vi "Kontrola poprawnego zakresu współrzędnej.vi"(8 "Sekundy":dbl, 9 "Minuty":dbl, 10 "Stopnie":dbl, 11 "Format współrzędnych":u16(ring) items=["D", "DM", "DMS"]) -> (0 "error constant":errorcluster)   [LabVIEW 2012, in "Biblioteka moduł map v3.lvlib" / "Konwersja wsp.lvlib" / "Obsługa błędów.lvlib"]
doc: "SubVI ma za zadanie sprawdzić poprawność zakresu wpisanych stopni, minut i sekund. Oraz czy nie wpisano dodatkowo minut i sekund, gdy wpisano maksymalną wartość stopni."
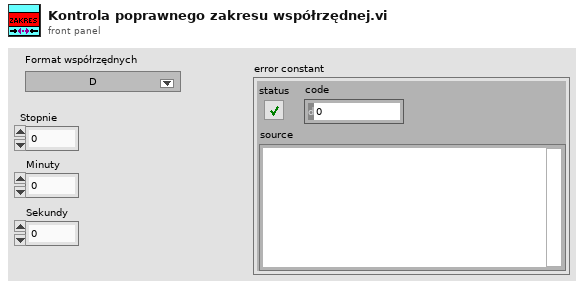
[diagram p1: front panel]
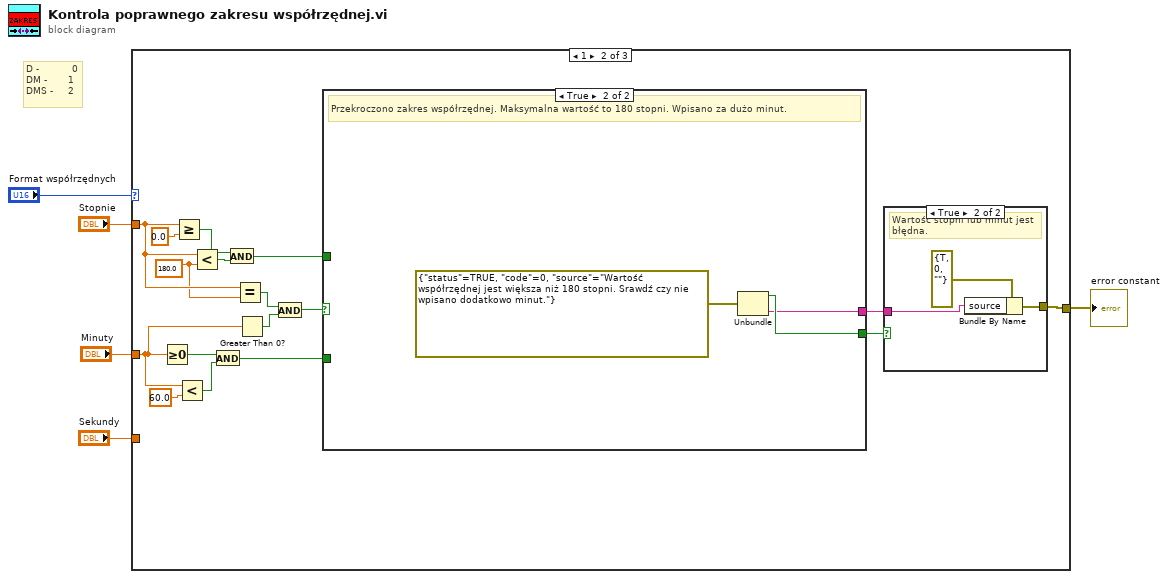
[diagram p0: block diagram]
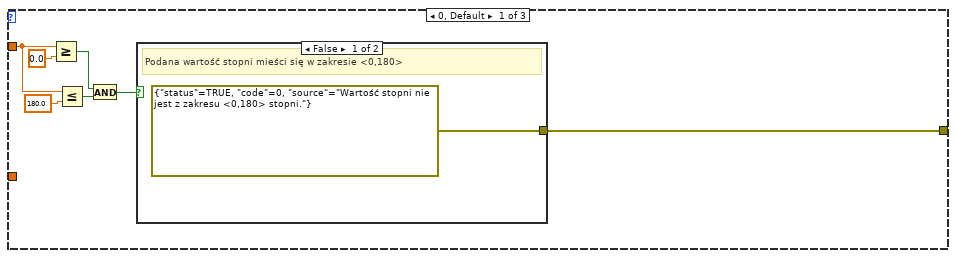
[diagram p2: hidden frame]
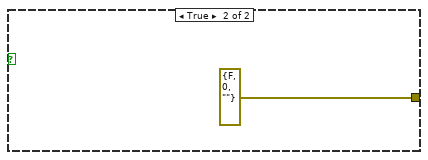
[diagram p3: hidden frame]
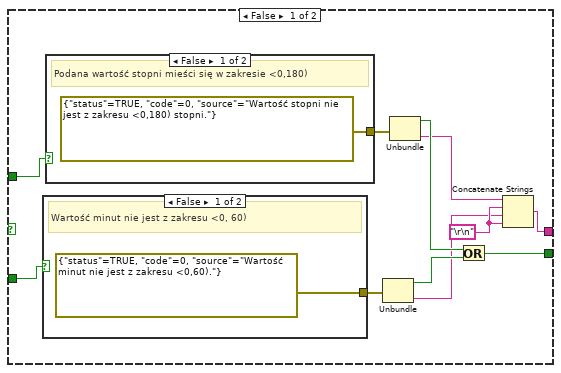
[diagram p4: hidden frame]
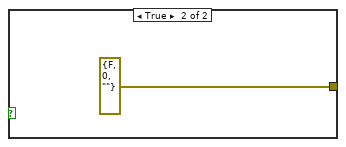
[diagram p5: hidden frame]
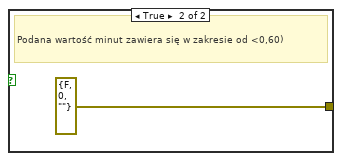
[diagram p6: hidden frame]
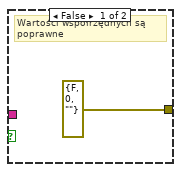
[diagram p7: hidden frame]
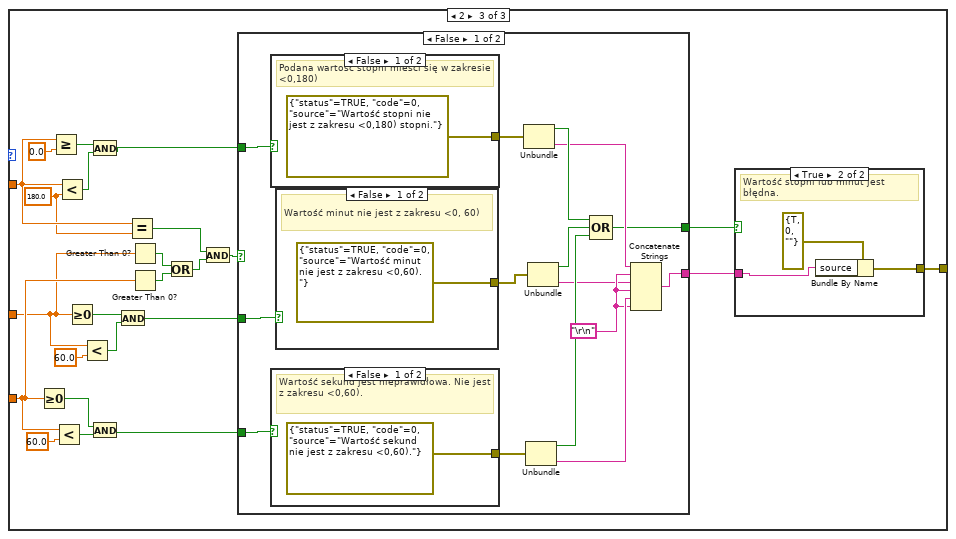
[diagram p8: hidden frame]
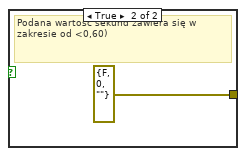
[diagram p9: hidden frame]
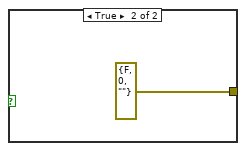
[diagram p10: hidden frame]
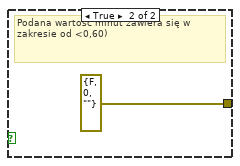
[diagram p11: hidden frame]
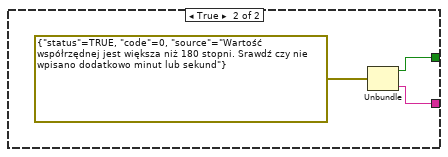
[diagram p12: hidden frame]
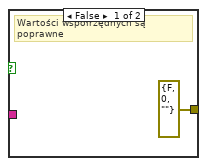
[diagram p13: hidden frame]
diagram:
  # "D -           0\nDM -       1\nDMS -     2"
  n1 = case shown="1" "Format współrzędnych" {
    tunnel: "Stopnie" -> [w8 w24 w60]
    tunnel: [w6 w26 w69] -> w1
    tunnel: "Minuty" -> [_ w22 w61]
    tunnel: "Sekundy" -> [_ _ w62]
    frame 0, Default {
      n2 = Greater Or Equal?(x=w8, y=0.0) -> (x >= y?=w11:bool)
      n3 = Less Or Equal?(x=w8, y=sgl 180.0) -> (x <= y?=w9:bool)
      n4 = And(x=w11, y=w9) -> (x .and. y?=w10:bool)
      n5 = case shown="False" w10 {
        tunnel: [errorcluster {"status"=TRUE, "code"=0, "source"="Wartość stopni nie jest z zakresu <0,180> stopni."} ("error constant") errorcluster {"status"=FALSE, "code"=0, "source"=""} ("error constant")] -> w6
        frame False {
          # "Podana wartość stopni mieści się w zakresie <0,180>"
        }
        frame True {
        }
      }
    }
    frame 1 {
      w23 = sgl 180.0 ("y")
      n6 = Greater Or Equal To 0?(x=w22) -> (x >= 0?=w25:bool)
      n7 = Greater Or Equal?(x=w24, y=0.0) -> (x >= y?=w28:bool)
      n8 = Less?(x=w22, y=sgl 60.0) -> (x < y?=w31:bool)
      n9 = Less?(x=w24, y=w23) -> (x < y?=w27:bool)
      n10 = And(x=w25, y=w31) -> (x .and. y?=w15:bool)
      n11 = And(x=w28, y=w27) -> (x .and. y?=w16:bool)
      n12 = Equal?(x=w24, y=w23) -> (x = y?=w20:bool)
      n13 = Greater Than 0?(x=w22) -> (x > 0?=w21:bool)
      n14 = And(x=w20, y=w21) -> (x .and. y?=w19:bool)
      n15 = case shown="True" w19 {
        tunnel: [w35 w47] -> w18
        tunnel: [w34 w48] -> w17
        tunnel: w16 -> [w33 _]
        tunnel: w15 -> [w32 _]
        frame False {
          w40 = "\r\n"
          n16 = case shown="False" w32 {
            tunnel: [errorcluster {"status"=TRUE, "code"=0, "source"="Wartość minut nie jest z zakresu <0,60)."} ("error constant") errorcluster {"status"=FALSE, "code"=0, "source"=""} ("error constant")] -> w36
            frame False {
              # "Wartość minut nie jest z zakresu <0, 60)"
            }
            frame True {
              # "Podana wartość minut zawiera się w zakresie od <0,60)"
            }
          }
          n17 = case shown="False" w33 {
            tunnel: [errorcluster {"status"=TRUE, "code"=0, "source"="Wartość stopni nie jest z zakresu <0,180) stopni."} ("error constant") errorcluster {"status"=FALSE, "code"=0, "source"=""} ("error constant")] -> w37
            frame False {
              # "Podana wartość stopni mieści się w zakresie <0,180)"
            }
            frame True {
            }
          }
          n18 = Unbundle(w36) -> ("status"=w41:bool, "source"=w39:string)  [unwired: 1 out]
          n19 = Unbundle(w37) -> ("status"=w42:bool, "source"=w38:string)  [unwired: 1 out]
          n20 = Or(x=w42, y=w41) -> (x .or. y?=w34:bool)
          n21 = Concatenate Strings(w38, w40, w39, w40) -> (w35:string)
        }
        frame True {
          # "Przekroczono zakres współrzędnej. Maksymalna wartość to 180 stopni. Wpisano za dużo minut."
          n22 = Unbundle(errorcluster {"status"=TRUE, "code"=0, "source"="Wartość współrzędnej jest większa niż 180 stopni. Srawdź czy nie wpisano dodatkowo minut."} ("error constant")) -> ("status"=w48:bool, "source"=w47:string)  [unwired: 1 out]
        }
      }
      n23 = case shown="True" w17 {
        tunnel: w18 -> [_ w52]
        tunnel: [errorcluster {"status"=FALSE, "code"=0, "source"=""} ("error constant") w51] -> w26
        frame False {
          # "Wartości współrzędnych są poprawne"
        }
        frame True {
          # "Wartość stopni lub minut jest błędna."
          n24 = Bundle By Name(cluster=errorcluster {"status"=TRUE, "code"=0, "source"=""} ("error constant"), "source"=w52) -> (w51:errorcluster)
        }
      }
    }
    frame 2 {
      w59 = sgl 180.0 ("y")
      n25 = Greater Or Equal To 0?(x=w62) -> (x >= 0?=w71:bool)
      n26 = Greater Or Equal?(x=w60, y=0.0) -> (x >= y?=w73:bool)
      n27 = Less?(x=w62, y=sgl 60.0) -> (x < y?=w70:bool)
      n28 = Less?(x=w60, y=w59) -> (x < y?=w68:bool)
      n29 = Greater Or Equal To 0?(x=w61) -> (x >= 0?=w76:bool)
      n30 = Less?(x=w61, y=sgl 60.0) -> (x < y?=w77:bool)
      n31 = And(x=w73, y=w68) -> (x .and. y?=w65:bool)
      n32 = And(x=w71, y=w70) -> (x .and. y?=w63:bool)
      n33 = And(x=w76, y=w77) -> (x .and. y?=w64:bool)
      n34 = Equal?(x=w60, y=w59) -> (x = y?=w55:bool)
      n35 = Greater Than 0?(x=w61) -> (x > 0?=w57:bool)
      n36 = Greater Than 0?(x=w62) -> (x > 0?=w58:bool)
      n37 = Or(x=w57, y=w58) -> (x .or. y?=w54:bool)
      n38 = And(x=w55, y=w54) -> (x .and. y?=w56:bool)
      n39 = case shown="False" w56 {
        tunnel: [w82 w99] -> w67
        tunnel: [w81 w100] -> w66
        tunnel: w65 -> [w80 _]
        tunnel: w64 -> [w79 _]
        tunnel: w63 -> [w78 _]
        frame False {
          w87 = "\r\n"
          n40 = case shown="False" w80 {
            tunnel: [errorcluster {"status"=TRUE, "code"=0, "source"="Wartość stopni nie jest z zakresu <0,180) stopni."} ("error constant") errorcluster {"status"=FALSE, "code"=0, "source"=""} ("error constant")] -> w84
            frame False {
              # "Podana wartość stopni mieści się w zakresie <0,180)"
            }
            frame True {
            }
          }
          n41 = case shown="False" w78 {
            tunnel: [errorcluster {"status"=TRUE, "code"=0, "source"="Wartość sekund nie jest z zakresu <0,60)."} ("error constant") errorcluster {"status"=FALSE, "code"=0, "source"=""} ("error constant")] -> w88
            frame False {
              # "Wartość sekund jest nieprawidłowa. Nie jest z zakresu <0,60)."
            }
            frame True {
              # "Podana wartość sekund zawiera się w zakresie od <0,60)"
            }
          }
          n42 = case shown="False" w79 {
            tunnel: [errorcluster {"status"=TRUE, "code"=0, "source"="Wartość minut nie jest z zakresu <0,60)."} ("error constant") errorcluster {"status"=FALSE, "code"=0, "source"=""} ("error constant")] -> w83
            frame False {
              # "Wartość minut nie jest z zakresu <0, 60)"
            }
            frame True {
              # "Podana wartość minut zawiera się w zakresie od <0,60)"
            }
          }
          n43 = Unbundle(w84) -> ("status"=w90:bool, "source"=w85:string)  [unwired: 1 out]
          n44 = Unbundle(w88) -> ("status"=w92:bool, "source"=w89:string)  [unwired: 1 out]
          n45 = Unbundle(w83) -> ("status"=w91:bool, "source"=w86:string)  [unwired: 1 out]
          n46 = Compound Arithmetic op=OR(w90, w91, w92) -> (w82:bool)
          n47 = Concatenate Strings(w85, w87, w86, w87, w89, w87) -> (w81:string)
        }
        frame True {
          n48 = Unbundle(errorcluster {"status"=TRUE, "code"=0, "source"="Wartość współrzędnej jest większa niż 180 stopni. Srawdź czy nie wpisano dodatkowo minut lub sekund"} ("error constant")) -> ("status"=w99:bool, "source"=w100:string)  [unwired: 1 out]
        }
      }
      n49 = case shown="True" w67 {
        tunnel: w66 -> [_ w104]
        tunnel: [errorcluster {"status"=FALSE, "code"=0, "source"=""} ("error constant") w103] -> w69
        frame False {
          # "Wartości współrzędnych są poprawne"
        }
        frame True {
          # "Wartość stopni lub minut jest błędna."
          n50 = Bundle By Name(cluster=errorcluster {"status"=TRUE, "code"=0, "source"=""} ("error constant"), "source"=w104) -> (w103:errorcluster)
        }
      }
    }
  }
  "error constant" <- w1
